vi "Handle Button Press.vi"(8 "error in (no error)":errorcluster, 10 "CtlRef":refnum<vi>, 11 "IDialogBox In":refnum<class "IDialogBox.lvclass">) -> (0 "error out":errorcluster, 3 "IDialogBox Out":refnum<class "IDialogBox.lvclass">)   [LabVIEW 2015, in "IDialogBox.lvlib" / "IDialogBox.lvclass"]
uses:
  IDialogBox.lvclass
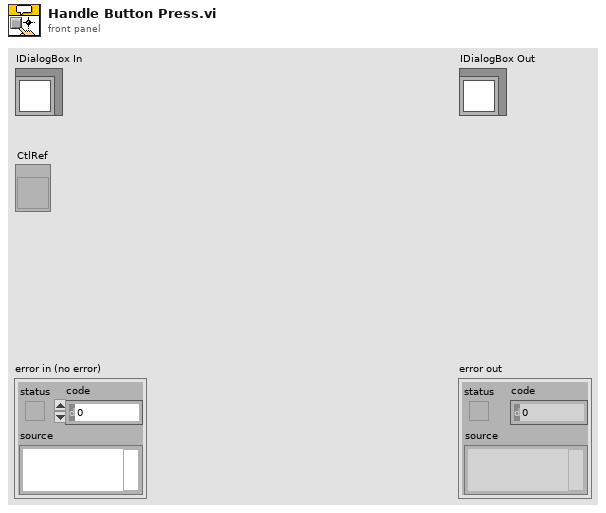
[diagram p1: front panel]
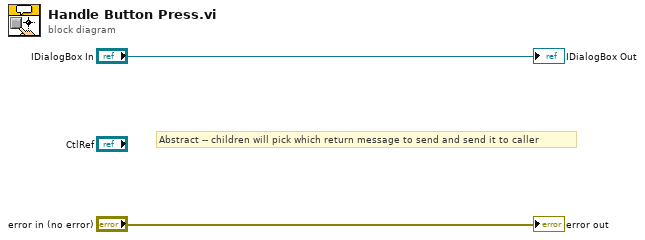
[diagram p0: block diagram]
diagram:
  # "Abstract -- children will pick which return message to send and send it to caller"
  "error out" <- "error in (no error)"
  "IDialogBox Out" <- "IDialogBox In"
